vi "AutoRun.vi"() -> ()   [LabVIEW 2013]
uses:
  resultShow.vi
panel:
  in  "布尔":bool
  out "毫秒计时值":u32
  in  "stepMotor/ECU":string
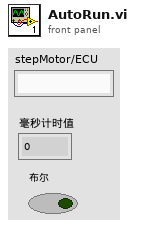
[diagram p1: front panel]
types:
  T1 = cluster{"takesTime":refnum<vi>, "userStatus":refnum<vi>, "userName":refnum<vi>, "connectionMode":refnum<vi>, "productsName":refnum<vi>, "rigStatus":refnum<vi>, "管柱码":refnum<vi>, "上序状态":refnum<vi>}
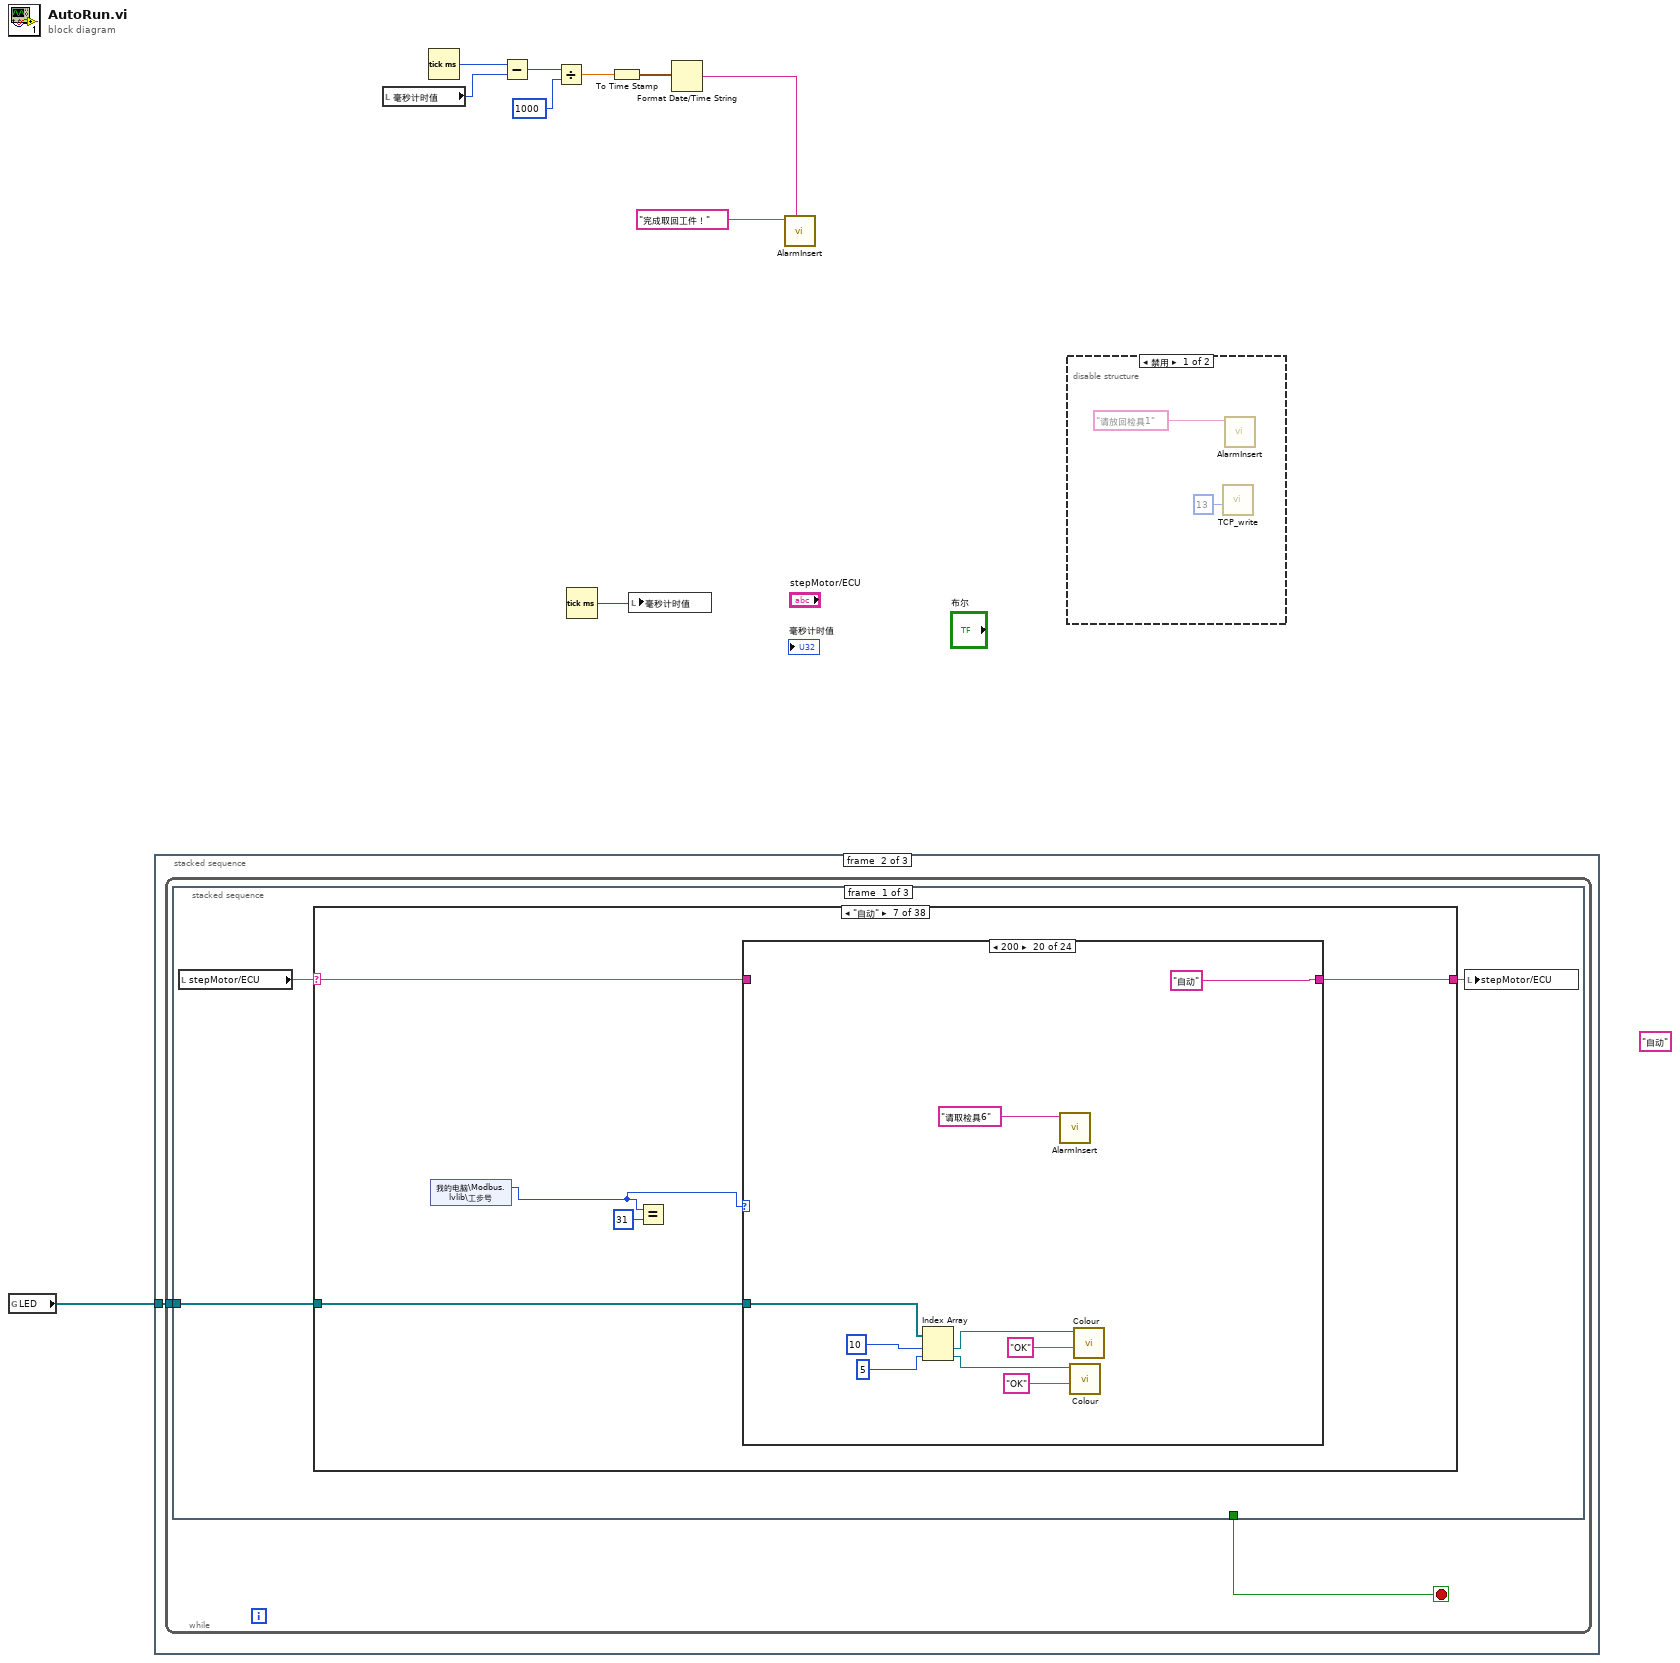
[diagram p0: block diagram]
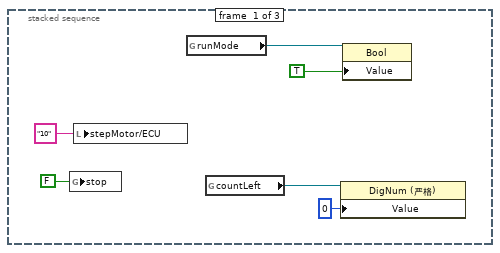
[diagram p3: hidden frame]
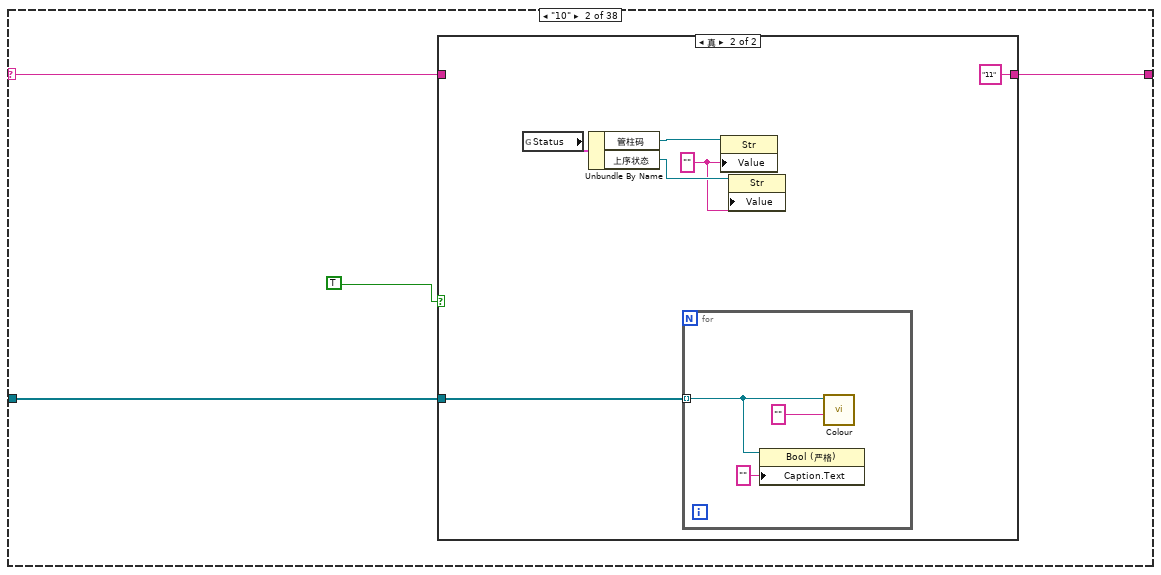
[diagram p5: hidden frame]
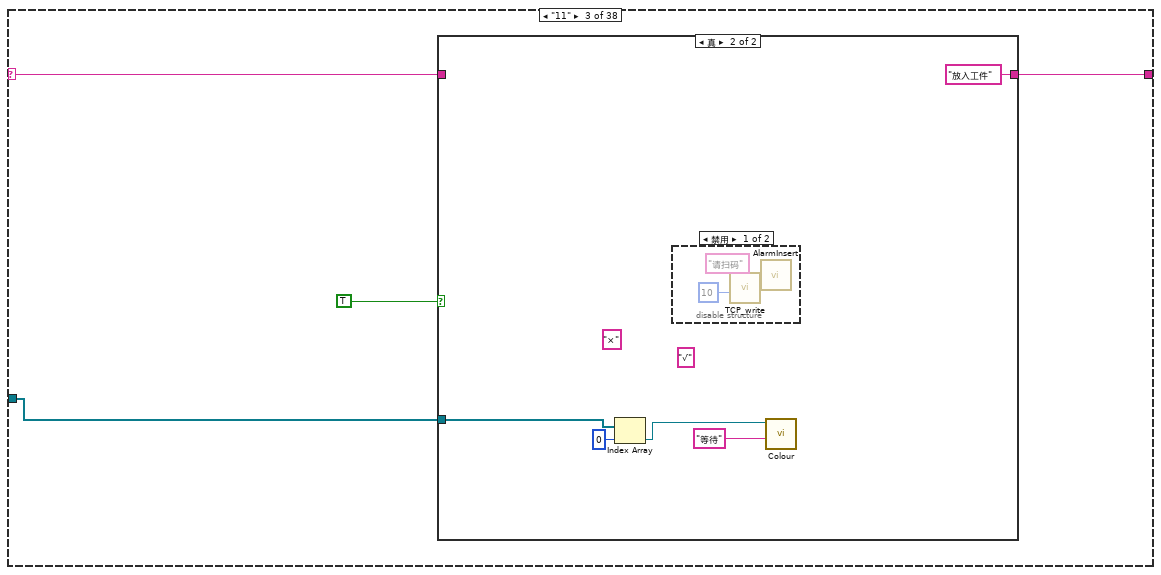
[diagram p7: hidden frame]
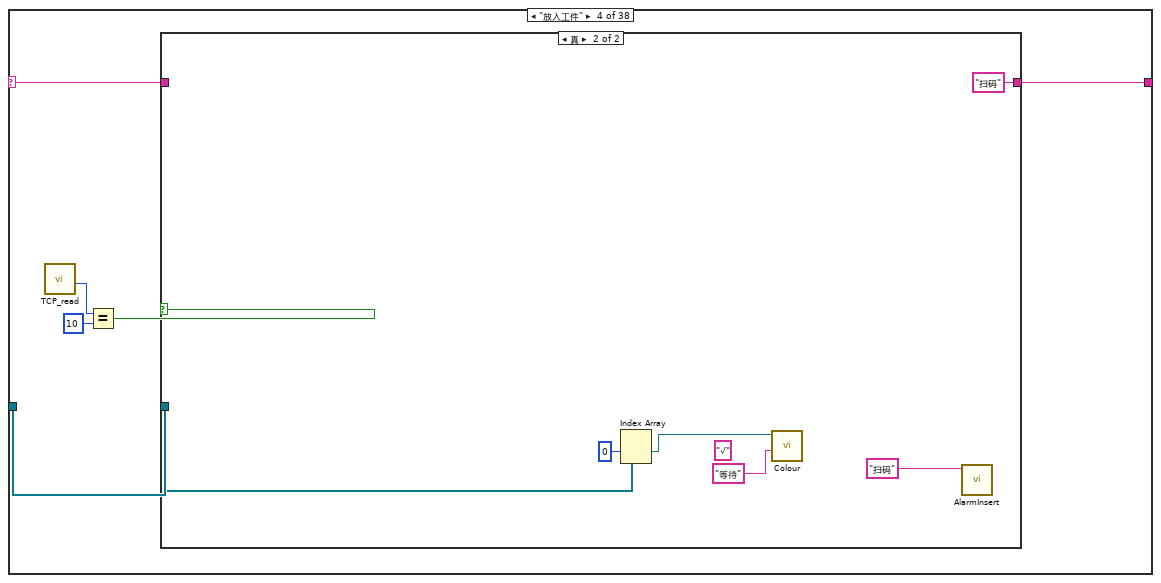
[diagram p10: hidden frame]
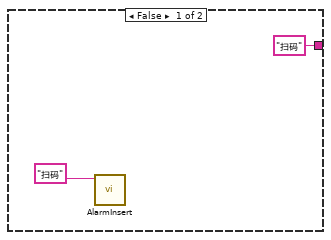
[diagram p11: hidden frame]
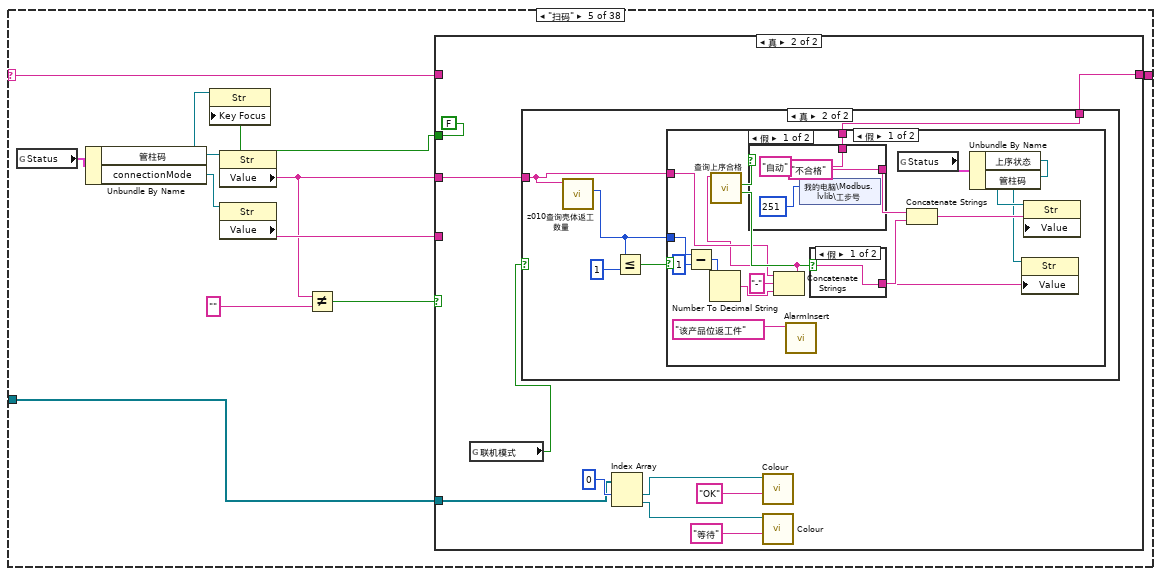
[diagram p12: hidden frame]
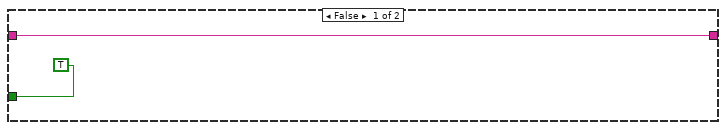
[diagram p13: hidden frame]
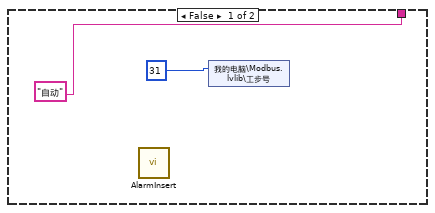
[diagram p14: hidden frame]
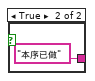
[diagram p15: hidden frame]
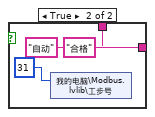
[diagram p16: hidden frame]
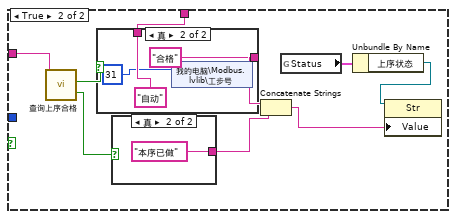
[diagram p17: hidden frame]
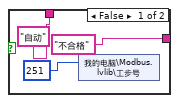
[diagram p19: hidden frame]
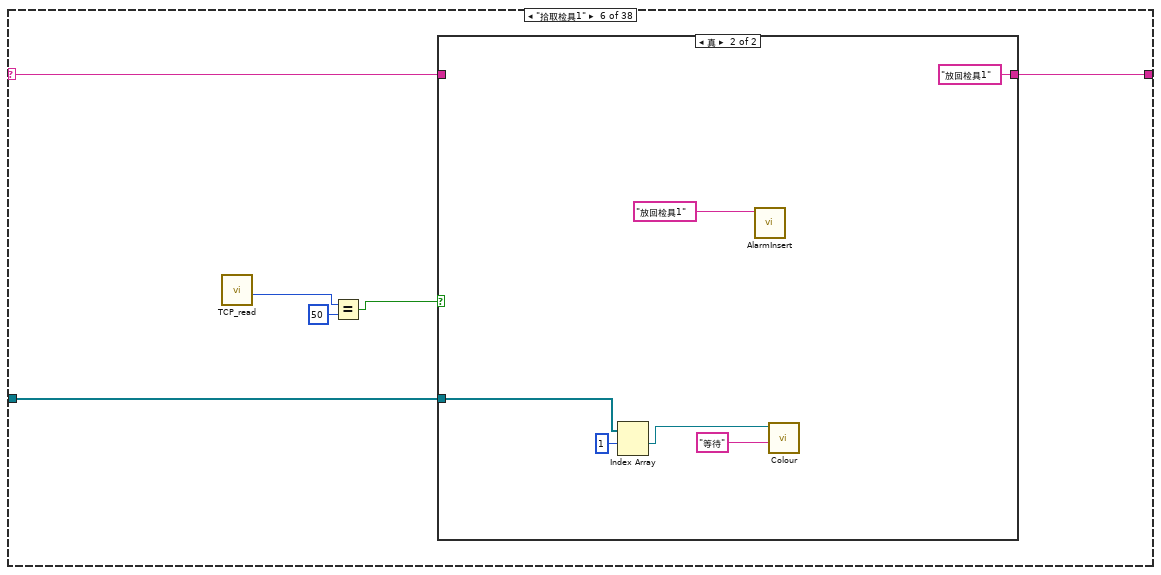
[diagram p20: hidden frame]
diagram:
  (unwired) "自动"
  n1 = global read "resultShow.vi" "LED"() -> (w10:refnum<vi>[])
  n2 = stacked-sequence {
    tunnel: w10 -> [_ w17 _]
    frame #0 {
      n3 = global write "全局 3.vi" "stop"(FALSE ("布尔 2")) -> ()
      n4 = local write "stepMotor/ECU"("10" ("step")) -> ()
      n5 = global read "resultShow.vi" "runMode"() -> (w13:refnum<vi>)
      n6 = global read "resultShow.vi" "countLeft"() -> (w11:refnum<vi>)
      n7 = property class="DigNum (严格)"(reference=w11, "Value"=u32 0 ("值")) -> ()  [unwired: 1 in, 2 out]
      n8 = property class="Bool"(reference=w13, "Value"=TRUE ("m")) -> ()  [unwired: 1 in, 2 out]
    }
    frame #1 {
      n9 = while {
        tunnel: w17 -> [w18]
        stop <- w19 stop-if-true
        n10 = stacked-sequence {
          tunnel: [_ _ w860] -> w19
          tunnel: w18 -> [w21 _ _]
          frame #0 {
            n11 = local read "stepMotor/ECU"() -> (w20:string)
            n12 = case shown="\"自动\"" w20 {
              selector: w20 -> [w23 w26 w40 w51 w72 w137 w149 w331 w347 w363 w381 w397 w413 w429 w445 w461 w477 w493 w509 w525 w541 w557 w573 w589 w605 w621 w637 w653 w669 w685 w701 w717 w733 w749 w765 w781 w795 w823]
              tunnel: [w23 w27 w41 w49 w71 w138 w150 w329 w345 w361 w382 w398 w414 w430 w446 w462 w478 w494 w510 w526 w542 w558 w574 w590 w606 w622 w638 w654 w670 w686 w702 w718 w734 w750 w766 w782 w796 w824] -> w22
              tunnel: w21 -> [_ w25 w39 w50 w73 w133 w147 w330 w346 w362 w377 w393 w409 w425 w441 w457 w473 w489 w505 w521 w537 w553 w569 w585 w601 w617 w633 w649 w665 w681 w697 w713 w729 w745 w761 w777 w794 w819]
              frame "假", Default {
              }
              frame "10" {
                n13 = case shown="真" TRUE {
                  tunnel: [w28 "11"] -> w27
                  tunnel: w26 -> [w28 _]
                  tunnel: w25 -> [_ w33]
                  frame False {
                  }
                  frame True {
                    w29 = ""
                    n14 = global read "resultShow.vi" "Status"() -> (w32:T1)
                    n15 = Unbundle By Name(w32) -> ("管柱码"=w31:refnum<vi>, "上序状态"=w30:refnum<vi>)
                    n16 = for {
                      tunnel: w33 -> [w36] mode=indexing
                      n17 = property class="Bool (严格)"(reference=w36, "Caption.Text"="" ("标题.文本")) -> ()  [unwired: 1 in, 2 out]
                      n18 = call "Colour.vi"("result"="" ("元素"), "colourRef"=w36) -> ()  [unwired: 9 in, 1 out]
                    }
                    n19 = property class="Str"(reference=w31, "Value"=w29) -> ()  [unwired: 1 in, 2 out]
                    n20 = property class="Str"(reference=w30, "Value"=w29) -> ()  [unwired: 1 in, 2 out]
                  }
                }
              }
              frame "11" {
                n21 = case shown="真" TRUE {
                  tunnel: [w42 "放入工件"] -> w41
                  tunnel: w40 -> [w42 _]
                  tunnel: w39 -> [_ w43]
                  frame False {
                  }
                  frame True {
                    (unwired) "×" ("元素")
                    (unwired) "√" ("元素")
                    n22 = Index Array(array=w43, index=0 ("索引")) -> (element=w45:refnum<vi>)
                    n23 = disable-structure shown="禁用" {
                      frame Disabled {
                        (unwired) "请扫码" ("消息名")
                        n24 = call "TCP_write.vi"("写入数据"=i8 10) -> ()  [unwired: 11 in]
                        n25 = call "AlarmInsert.vi"() -> ()  [unwired: 12 in]
                      }
                      frame Enabled {
                      }
                    }
                    n26 = call "Colour.vi"("result"="等待" ("元素"), "colourRef"=w45) -> ()  [unwired: 9 in, 1 out]
                  }
                }
              }
              frame "放入工件" {
                n27 = call "TCP_read.vi"() -> ("元素"=w52:u8)  [unwired: 10 in, 1 out]
                n28 = Equal?(x=w52, y=i8 10) -> (x = y?=w54:bool)
                n29 = case shown="真" w54 {
                  tunnel: ["扫码" "扫码"] -> w49
                  tunnel: w51 -> [_ _]
                  tunnel: w50 -> [_ w59]
                  frame False {
                    n30 = call "AlarmInsert.vi"("消息名"="扫码" ("string_5")) -> ()  [unwired: 11 in]
                  }
                  frame True {
                    (unwired) "√" ("元素")
                    n31 = Index Array(array=w59, index #1=0 ("索引")) -> (element #1=w61:refnum<vi>)  [unwired: 1 in, 1 out]
                    n32 = call "Colour.vi"("result"="等待" ("元素"), "colourRef"=w61) -> ()  [unwired: 9 in, 1 out]
                    n33 = call "AlarmInsert.vi"("消息名"="扫码" ("string_5")) -> ()  [unwired: 11 in]
                  }
                }
              }
              frame "扫码" {
                n34 = global read "resultShow.vi" "Status"() -> (w70:T1)
                n35 = Unbundle By Name(w70) -> ("管柱码"=w68:refnum<vi>, "connectionMode"=w65:refnum<vi>)
                n36 = property class="Str"(reference=w68) -> ("Value"=w63:string)  [unwired: 1 in, 2 out]
                n37 = property class="Str"(reference=w65) -> ("Value"=w64:string)  [unwired: 1 in, 2 out]
                n38 = Not Equal?(x=w63, y="") -> (x != y?=w67:bool)
                n39 = case shown="真" w67 {
                  tunnel: [w75 w76] -> w71
                  tunnel: w72 -> [w75 _]
                  tunnel: w73 -> [_ w82]
                  tunnel: [TRUE FALSE] -> w66
                  tunnel: w64 -> [_ _]
                  tunnel: w63 -> [_ w78]
                  frame False {
                  }
                  frame True {
                    n40 = global read "resultShow.vi" "联机模式"() -> (w77:bool)
                    n41 = case shown="真" w77 {
                      tunnel: w78 -> [_ w90]
                      tunnel: ["自动" ("消息名") w88] -> w76
                      frame False {
                        n42 = call "AlarmInsert.vi"() -> ()  [unwired: 12 in]
                        n43 = shared-variable "我的电脑\\Modbus.lvlib\\工步号"(i8 31 ("写入数据")) -> ()  [unwired: 1 in, 1 out]
                      }
                      frame True {
                        n44 = call "z010查询壳体返工数量.vi"("转向器总成ID"=w90) -> ("Rows Fetched"=w89:i32)  [unwired: 8 in, 2 out]
                        n45 = Less Or Equal?(x=w89, y=1) -> (x <= y?=w91:bool)
                        n46 = case shown="假" w91 {
                          tunnel: w90 -> [w96 w125]
                          tunnel: w89 -> [w101 _]
                          tunnel: [w93 w117] -> w88
                          frame False {
                            n47 = Subtract(x=w101, y=1) -> (x-y=w99:i32)
                            n48 = Number To Decimal String ("数值至十进制数字符串转换")(number=w99) -> (decimal integer string=w98:string)  [unwired: 1 in]
                            n49 = Concatenate Strings(w96, "-" ("字符串"), w98) -> (w94:string)
                            n50 = call "查询上序合格.vi"("产品ID"=w94) -> ("本序已做"=w107:bool, "上序合格"=w108:bool)  [unwired: 8 in, 1 out]
                            n51 = case shown="假" w108 {
                              tunnel: ["不合格" "合格"] -> w104
                              tunnel: ["自动" ("string_5") "自动"] -> w93
                              frame False {
                                n52 = shared-variable "我的电脑\\Modbus.lvlib\\工步号"(251 ("写入数据")) -> ()  [unwired: 1 in, 1 out]
                              }
                              frame True {
                                n53 = shared-variable "我的电脑\\Modbus.lvlib\\工步号"(i8 31 ("写入数据")) -> ()  [unwired: 1 in, 1 out]
                              }
                            }
                            n54 = call "AlarmInsert.vi"("消息名"="该产品位返工件") -> ()  [unwired: 11 in]
                            n55 = case shown="假" w107 {
                              tunnel: [_ "本序已做"] -> w103
                              frame False {
                              }
                              frame True {
                              }
                            }
                            n56 = global read "resultShow.vi" "Status"() -> (w106:T1)
                            n57 = Concatenate Strings(w104, w103) -> (w102:string)
                            n58 = Unbundle By Name(w106) -> ("上序状态"=w105:refnum<vi>, "管柱码"=w95:refnum<vi>)
                            n59 = property class="Str"(reference=w95, "Value"=w94) -> ()  [unwired: 1 in, 2 out]
                            n60 = property class="Str"(reference=w105, "Value"=w102) -> ()  [unwired: 1 in, 2 out]
                          }
                          frame True {
                            n61 = call "查询上序合格.vi"("产品ID"=w125) -> ("本序已做"=w123:bool, "上序合格"=w124:bool)  [unwired: 8 in, 1 out]
                            n62 = case shown="真" w124 {
                              tunnel: ["不合格" "合格"] -> w120
                              tunnel: ["自动" "自动" ("string_5")] -> w117
                              frame False {
                                n63 = shared-variable "我的电脑\\Modbus.lvlib\\工步号"(251 ("索引")) -> ()  [unwired: 1 in, 1 out]
                              }
                              frame True {
                                n64 = shared-variable "我的电脑\\Modbus.lvlib\\工步号"(i8 31 ("写入数据")) -> ()  [unwired: 1 in, 1 out]
                              }
                            }
                            n65 = case shown="真" w123 {
                              tunnel: [_ "本序已做"] -> w119
                              frame False {
                              }
                              frame True {
                              }
                            }
                            n66 = Concatenate Strings(w120, w119) -> (w118:string)
                            n67 = global read "resultShow.vi" "Status"() -> (w122:T1)
                            n68 = Unbundle By Name(w122) -> ("上序状态"=w121:refnum<vi>)
                            n69 = property class="Str"(reference=w121, "Value"=w118) -> ()  [unwired: 1 in, 2 out]
                          }
                        }
                      }
                    }
                    n70 = Index Array(array=w82, index #1=0 ("索引")) -> (element #1=w84:refnum<vi>, element #2=w80:refnum<vi>)  [unwired: 1 in]
                    n71 = call "Colour.vi"("result"="OK" ("元素"), "colourRef"=w84) -> ()  [unwired: 9 in, 1 out]
                    n72 = call "Colour.vi"("result"="等待" ("元素"), "colourRef"=w80) -> ()  [unwired: 9 in, 1 out]
                  }
                }
                n73 = property class="Str"(reference=w68, "Key Focus"=w66) -> ()  [unwired: 1 in, 2 out]
              }
              frame "拾取检具1" {
                n74 = call "TCP_read.vi"() -> ("元素"=w136:u8)  [unwired: 10 in, 1 out]
                n75 = Equal?(x=w136, y=i8 50) -> (x = y?=w134:bool)
                n76 = case shown="真" w134 {
                  tunnel: [w139 "放回检具1"] -> w138
                  tunnel: w137 -> [w139 _]
                  tunnel: w133 -> [_ w141]
                  frame False {
                  }
                  frame True {
                    n77 = Index Array(array=w141, index #1=1 ("索引")) -> (element #1=w143:refnum<vi>)  [unwired: 1 in, 1 out]
                    n78 = call "AlarmInsert.vi"("消息名"="放回检具1" ("string_5")) -> ()  [unwired: 11 in]
                    n79 = call "Colour.vi"("result"="等待" ("元素"), "colourRef"=w143) -> ()  [unwired: 9 in, 1 out]
                  }
                }
              }
              frame "自动" {
                n80 = shared-variable "我的电脑\\Modbus.lvlib\\工步号"() -> (w146:u16)  [unwired: 1 in, 1 out]
                n81 = Equal?(x=w146, y=i8 31) -> ()  [unwired: 1 out]
                n82 = case shown="200" w146 {
                  tunnel: ["自动" "自动" "自动" "自动" "自动" "自动" "自动" "自动" "自动" "自动" "自动" "自动" "自动" "自动" "自动" "自动" "自动" "自动" "自动" "自动" "自动" "10" w313 _] -> w150
                  tunnel: w149 -> [_ _ _ _ _ _ _ _ _ _ _ _ _ _ _ _ _ _ _ _ _ _ _ _]
                  tunnel: w147 -> [_ w154 w163 w172 w186 w189 w203 w211 w220 w226 w235 w240 w248 w254 w263 w272 w281 w287 w296 w305 w311 _ _ w328]
                  frame 0, Default {
                  }
                  frame 31 {
                    n83 = disable-structure shown="禁用" {
                      disable-tunnel: w154 -> [w155 _]
                      frame Disabled {
                        n84 = Index Array(array=w155, index #1=1 ("索引")) -> (element #1=w159:refnum<vi>, element #2=w156:refnum<vi>)  [unwired: 1 in]
                        n85 = call "Colour.vi"("result"="√" ("元素"), "colourRef"=w159) -> ()  [unwired: 9 in, 1 out]
                        n86 = call "Colour.vi"("result"="×" ("元素"), "colourRef"=w156) -> ()  [unwired: 9 in, 1 out]
                      }
                      frame Enabled {
                      }
                    }
                    n87 = call "AlarmInsert.vi"("消息名"="请检查左右拉杆是否在位" ("string_5")) -> ()  [unwired: 11 in]
                  }
                  frame 32 {
                    n88 = disable-structure shown="禁用" {
                      disable-tunnel: w163 -> [w164 _]
                      frame Disabled {
                        n89 = Index Array(array=w164, index #1=1 ("索引")) -> (element #1=w168:refnum<vi>, element #2=w165:refnum<vi>)  [unwired: 1 in]
                        n90 = call "Colour.vi"("result"="√" ("元素"), "colourRef"=w168) -> ()  [unwired: 9 in, 1 out]
                        n91 = call "Colour.vi"("result"="×" ("元素"), "colourRef"=w165) -> ()  [unwired: 9 in, 1 out]
                      }
                      frame Enabled {
                      }
                    }
                    n92 = call "AlarmInsert.vi"("消息名"="请按启动按钮开始" ("string_5")) -> ()  [unwired: 11 in]
                  }
                  frame 33 {
                    n93 = disable-structure shown="禁用" {
                      disable-tunnel: w172 -> [w173 _]
                      frame Disabled {
                        n94 = Index Array(array=w173, index #1=1 ("索引")) -> (element #1=w177:refnum<vi>, element #2=w174:refnum<vi>)  [unwired: 1 in]
                        n95 = call "Colour.vi"("result"="√" ("元素"), "colourRef"=w177) -> ()  [unwired: 9 in, 1 out]
                        n96 = call "Colour.vi"("result"="×" ("元素"), "colourRef"=w174) -> ()  [unwired: 9 in, 1 out]
                      }
                      frame Enabled {
                      }
                    }
                    n97 = call "AlarmInsert.vi"("消息名"="气缸进" ("string_5")) -> ()  [unwired: 11 in]
                  }
                  frame 50 {
                    n98 = Index Array(array=w186, index #1=1 ("索引")) -> (element #1=w183:refnum<vi>, element #2=w180:refnum<vi>)  [unwired: 1 in]
                    n99 = call "AlarmInsert.vi"("消息名"="请取检具1" ("string_5")) -> ()  [unwired: 11 in]
                    n100 = call "Colour.vi"("result"="等待" ("元素"), "colourRef"=w183) -> ()  [unwired: 9 in, 1 out]
                    n101 = call "Colour.vi"("result"="×" ("元素"), "colourRef"=w180) -> ()  [unwired: 9 in, 1 out]
                  }
                  frame 60 {
                    n102 = disable-structure shown="禁用" {
                      disable-tunnel: w189 -> [w195 _]
                      frame Disabled {
                        n103 = Index Array(array=w195, index #1=1 ("索引")) -> (element #1=w193:refnum<vi>, element #2=w190:refnum<vi>)  [unwired: 1 in]
                        n104 = call "Colour.vi"("result"="等待" ("元素"), "colourRef"=w193) -> ()  [unwired: 9 in, 1 out]
                        n105 = call "Colour.vi"("result"="×" ("元素"), "colourRef"=w190) -> ()  [unwired: 9 in, 1 out]
                      }
                      frame Enabled {
                      }
                    }
                    n106 = call "AlarmInsert.vi"("消息名"="请放回检具1" ("string_5")) -> ()  [unwired: 11 in]
                  }
                  frame 70 {
                    n107 = Index Array(array=w203, index #1=1 ("索引")) -> (element #1=w200:refnum<vi>, element #2=w197:refnum<vi>)  [unwired: 1 in]
                    n108 = call "AlarmInsert.vi"("消息名"="请取检具2" ("string_5")) -> ()  [unwired: 11 in]
                    n109 = call "Colour.vi"("result"="OK" ("元素"), "colourRef"=w200) -> ()  [unwired: 9 in, 1 out]
                    n110 = call "Colour.vi"("result"="等待" ("元素"), "colourRef"=w197) -> ()  [unwired: 9 in, 1 out]
                  }
                  frame 80 {
                    n111 = Index Array(array=w211, index #1=1 ("索引")) -> (element #1=w208:refnum<vi>, element #2=w205:refnum<vi>)  [unwired: 1 in]
                    n112 = call "AlarmInsert.vi"("消息名"="请放回检具2" ("string_5")) -> ()  [unwired: 11 in]
                    n113 = call "Colour.vi"("result"="OK" ("元素"), "colourRef"=w208) -> ()  [unwired: 9 in, 1 out]
                    n114 = call "Colour.vi"("result"="等待" ("元素"), "colourRef"=w205) -> ()  [unwired: 9 in, 1 out]
                  }
                  frame 90 {
                    n115 = Index Array(array=w220, index #1=2 ("索引"), index #2=9 ("索引")) -> (element #1=w217:refnum<vi>, element #2=w214:refnum<vi>)
                    n116 = call "AlarmInsert.vi"("消息名"="请取检具9" ("string_5")) -> ()  [unwired: 11 in]
                    n117 = call "Colour.vi"("result"="OK" ("元素"), "colourRef"=w217) -> ()  [unwired: 9 in, 1 out]
                    n118 = call "Colour.vi"("result"="等待" ("元素"), "colourRef"=w214) -> ()  [unwired: 9 in, 1 out]
                  }
                  frame 100 {
                    n119 = Index Array(array=w226, index=9 ("索引")) -> (element=w223:refnum<vi>)
                    n120 = call "AlarmInsert.vi"("消息名"="请放回检具9" ("string_5")) -> ()  [unwired: 11 in]
                    n121 = call "Colour.vi"("result"="等待" ("元素"), "colourRef"=w223) -> ()  [unwired: 9 in, 1 out]
                  }
                  frame 110 {
                    n122 = Index Array(array=w235, index #1=9 ("索引"), index #2=3 ("索引")) -> (element #1=w232:refnum<vi>, element #2=w228:refnum<vi>)
                    n123 = call "AlarmInsert.vi"("消息名"="请取检具3" ("string_5")) -> ()  [unwired: 11 in]
                    n124 = call "Colour.vi"("result"="OK" ("元素"), "colourRef"=w232) -> ()  [unwired: 9 in, 1 out]
                    n125 = call "Colour.vi"("result"="等待" ("元素"), "colourRef"=w228) -> ()  [unwired: 9 in, 1 out]
                  }
                  frame 120 {
                    (unwired) "" ("元素")
                    n126 = Index Array(array=w240, index #1=3 ("索引"), index #2=3 ("索引")) -> ()  [unwired: 2 out]
                    n127 = call "AlarmInsert.vi"("消息名"="请放回检具3" ("string_5")) -> ()  [unwired: 11 in]
                  }
                  frame 130 {
                    n128 = Index Array(array=w248, index #1=3 ("索引")) -> (element #1=w245:refnum<vi>, element #2=w241:refnum<vi>)  [unwired: 1 in]
                    n129 = call "AlarmInsert.vi"("消息名"="请取检具4" ("string_5")) -> ()  [unwired: 11 in]
                    n130 = call "Colour.vi"("result"="OK" ("元素"), "colourRef"=w245) -> ()  [unwired: 9 in, 1 out]
                    n131 = call "Colour.vi"("result"="等待" ("元素"), "colourRef"=w241) -> ()  [unwired: 9 in, 1 out]
                  }
                  frame 140 {
                    n132 = Index Array(array=w254, index #1=4 ("索引")) -> (element #1=w251:refnum<vi>)  [unwired: 1 in, 1 out]
                    n133 = call "AlarmInsert.vi"("消息名"="请放回检具4" ("string_5")) -> ()  [unwired: 11 in]
                    n134 = call "Colour.vi"("result"="等待" ("元素"), "colourRef"=w251) -> ()  [unwired: 9 in, 1 out]
                  }
                  frame 150 {
                    n135 = Index Array(array=w263, index #1=4 ("索引"), index #2=5 ("索引")) -> (element #1=w260:refnum<vi>, element #2=w256:refnum<vi>)
                    n136 = call "AlarmInsert.vi"("消息名"="请取检具5" ("string_5")) -> ()  [unwired: 11 in]
                    n137 = call "Colour.vi"("result"="等待" ("元素"), "colourRef"=w256) -> ()  [unwired: 9 in, 1 out]
                    n138 = call "Colour.vi"("result"="OK" ("元素"), "colourRef"=w260) -> ()  [unwired: 9 in, 1 out]
                  }
                  frame 160 {
                    n139 = Index Array(array=w272, index #1=4 ("索引"), index #2=5 ("索引")) -> (element #1=w269:refnum<vi>, element #2=w265:refnum<vi>)
                    n140 = call "AlarmInsert.vi"("消息名"="请放回检具5" ("string_5")) -> ()  [unwired: 11 in]
                    n141 = call "Colour.vi"("result"="等待" ("元素"), "colourRef"=w265) -> ()  [unwired: 9 in, 1 out]
                    n142 = call "Colour.vi"("result"="OK" ("元素"), "colourRef"=w269) -> ()  [unwired: 9 in, 1 out]
                  }
                  frame 170 {
                    n143 = Index Array(array=w281, index #1=5 ("索引"), index #2=10 ("索引")) -> (element #1=w278:refnum<vi>, element #2=w274:refnum<vi>)
                    n144 = call "AlarmInsert.vi"("消息名"="请取检具10" ("string_5")) -> ()  [unwired: 11 in]
                    n145 = call "Colour.vi"("result"="等待" ("元素"), "colourRef"=w274) -> ()  [unwired: 9 in, 1 out]
                    n146 = call "Colour.vi"("result"="OK" ("元素"), "colourRef"=w278) -> ()  [unwired: 9 in, 1 out]
                  }
                  frame 180 {
                    n147 = Index Array(array=w287, index #1=10 ("索引")) -> (element #1=w284:refnum<vi>)  [unwired: 1 in, 1 out]
                    n148 = call "AlarmInsert.vi"("消息名"="请放回检具10" ("string_5")) -> ()  [unwired: 11 in]
                    n149 = call "Colour.vi"("result"="等待" ("元素"), "colourRef"=w284) -> ()  [unwired: 9 in, 1 out]
                  }
                  frame 190 {
                    n150 = Index Array(array=w296, index #1=10 ("索引"), index #2=5 ("索引")) -> (element #1=w293:refnum<vi>, element #2=w289:refnum<vi>)
                    n151 = call "AlarmInsert.vi"("消息名"="请取检具6" ("string_5")) -> ()  [unwired: 11 in]
                    n152 = call "Colour.vi"("result"="等待" ("元素"), "colourRef"=w289) -> ()  [unwired: 9 in, 1 out]
                    n153 = call "Colour.vi"("result"="OK" ("元素"), "colourRef"=w293) -> ()  [unwired: 9 in, 1 out]
                  }
                  frame 200 {
                    n154 = Index Array(array=w305, index #1=10 ("索引"), index #2=5 ("索引")) -> (element #1=w302:refnum<vi>, element #2=w298:refnum<vi>)
                    n155 = call "AlarmInsert.vi"("消息名"="请取检具6" ("string_5")) -> ()  [unwired: 11 in]
                    n156 = call "Colour.vi"("result"="OK" ("元素"), "colourRef"=w298) -> ()  [unwired: 9 in, 1 out]
                    n157 = call "Colour.vi"("result"="OK" ("元素"), "colourRef"=w302) -> ()  [unwired: 9 in, 1 out]
                  }
                  frame 210 {
                    n158 = Index Array(array=w311, index #1=5 ("索引"), index #2=5 ("索引")) -> (element #1=w309:refnum<vi>)  [unwired: 1 out]
                    n159 = call "Colour.vi"("result"="OK" ("元素"), "colourRef"=w309) -> ()  [unwired: 9 in, 1 out]
                  }
                  frame 251 {
                  }
                  frame 250 {
                    n160 = stacked-sequence {
                      tunnel: [_ "10"] -> w313
                      frame #0 {
                        w320 = "1"
                        n161 = global read "resultShow.vi" "Status"() -> (w319:T1)
                        n162 = Unbundle By Name(w319) -> ("管柱码"=w318:refnum<vi>, "userName"=w316:refnum<vi>)
                        n163 = property class="Str"(reference=w316) -> ("Value"=w315:string)  [unwired: 1 in, 2 out]
                        n164 = property class="Str"(reference=w318) -> ("Value"=w317:string)  [unwired: 1 in, 2 out]
                        n165 = Build Array(w317, w315, w320, w320) -> (w314:string[])
                        n166 = call "数据库更新.vi"("设备号"="14", "数据"=w314) -> ()  [unwired: 13 in, 1 out]
                      }
                      frame #1 {
                        n167 = shared-variable "我的电脑\\Modbus.lvlib\\工步号"(251) -> ()  [unwired: 1 in, 1 out]
                      }
                    }
                  }
                  frame 51 {
                    n168 = Index Array(array=w328, index=1 ("索引")) -> (element=w325:refnum<vi>)
                    n169 = call "AlarmInsert.vi"("消息名"="请取检具1" ("string_5")) -> ()  [unwired: 11 in]
                    n170 = call "Colour.vi"("result"="等待" ("元素"), "colourRef"=w325) -> ()  [unwired: 9 in, 1 out]
                  }
                }
              }
              frame "放回检具1" {
                n171 = call "TCP_read.vi"() -> ("元素"=w334:u8)  [unwired: 10 in, 1 out]
                n172 = Equal?(x=w334, y=i8 60) -> (x = y?=w332:bool)
                n173 = case shown="真" w332 {
                  tunnel: [w335 "拾取检具2"] -> w329
                  tunnel: w331 -> [w335 _]
                  tunnel: w330 -> [_ w337]
                  frame False {
                  }
                  frame True {
                    n174 = Index Array(array=w337, index #1=2 ("索引")) -> (element #1=w341:refnum<vi>, element #2=w338:refnum<vi>)  [unwired: 1 in]
                    n175 = call "TCP_write.vi"("写入数据"=i8 20) -> ()  [unwired: 11 in]
                    n176 = call "AlarmInsert.vi"("消息名"="拾取检具2" ("string_5")) -> ()  [unwired: 11 in]
                    n177 = call "Colour.vi"("result"="OK" ("元素"), "colourRef"=w341) -> ()  [unwired: 9 in, 1 out]
                    n178 = call "Colour.vi"("result"="等待" ("元素"), "colourRef"=w338) -> ()  [unwired: 9 in, 1 out]
                  }
                }
              }
              frame "拾取检具2" {
                n179 = call "TCP_read.vi"() -> ("元素"=w348:u8)  [unwired: 10 in, 1 out]
                n180 = Equal?(x=w348, y=i8 21) -> (x = y?=w350:bool)
                n181 = case shown="真" w350 {
                  tunnel: [w351 "放回检具2"] -> w345
                  tunnel: w347 -> [w351 _]
                  tunnel: w346 -> [_ w353]
                  frame False {
                  }
                  frame True {
                    n182 = Index Array(array=w353, index #1=2 ("索引")) -> (element #1=w357:refnum<vi>, element #2=w354:refnum<vi>)  [unwired: 1 in]
                    n183 = call "TCP_write.vi"("写入数据"=i8 23) -> ()  [unwired: 11 in]
                    n184 = call "AlarmInsert.vi"("消息名"="放回检具2" ("string_5")) -> ()  [unwired: 11 in]
                    n185 = call "Colour.vi"("result"="√" ("元素"), "colourRef"=w357) -> ()  [unwired: 9 in, 1 out]
                    n186 = call "Colour.vi"("result"="×" ("元素"), "colourRef"=w354) -> ()  [unwired: 9 in, 1 out]
                  }
                }
              }
              frame "放回检具2" {
                n187 = call "TCP_read.vi"() -> ("元素"=w364:u8)  [unwired: 10 in, 1 out]
                n188 = Equal?(x=w364, y=i8 25) -> (x = y?=w366:bool)
                n189 = case shown="真" w366 {
                  tunnel: [w367 "拾取检具3"] -> w361
                  tunnel: w363 -> [w367 _]
                  tunnel: w362 -> [_ w369]
                  frame False {
                  }
                  frame True {
                    n190 = Index Array(array=w369, index #1=3 ("索引")) -> (element #1=w373:refnum<vi>, element #2=w370:refnum<vi>)  [unwired: 1 in]
                    n191 = call "TCP_write.vi"("写入数据"=i8 30) -> ()  [unwired: 11 in]
                    n192 = call "AlarmInsert.vi"("消息名"="拾取检具3" ("string_5")) -> ()  [unwired: 11 in]
                    n193 = call "Colour.vi"("result"="√" ("元素"), "colourRef"=w373) -> ()  [unwired: 9 in, 1 out]
                    n194 = call "Colour.vi"("result"="×" ("元素"), "colourRef"=w370) -> ()  [unwired: 9 in, 1 out]
                  }
                }
              }
              frame "拾取检具3" {
                n195 = call "TCP_read.vi"() -> ("元素"=w380:u8)  [unwired: 10 in, 1 out]
                n196 = Equal?(x=w380, y=i8 31) -> (x = y?=w378:bool)
                n197 = case shown="真" w378 {
                  tunnel: [w383 "放回检具3"] -> w382
                  tunnel: w381 -> [w383 _]
                  tunnel: w377 -> [_ w385]
                  frame False {
                  }
                  frame True {
                    n198 = Index Array(array=w385, index #1=3 ("索引")) -> (element #1=w389:refnum<vi>, element #2=w386:refnum<vi>)  [unwired: 1 in]
                    n199 = call "TCP_write.vi"("写入数据"=i8 33) -> ()  [unwired: 11 in]
                    n200 = call "AlarmInsert.vi"("消息名"="放回检具3" ("string_5")) -> ()  [unwired: 11 in]
                    n201 = call "Colour.vi"("result"="√" ("元素"), "colourRef"=w389) -> ()  [unwired: 9 in, 1 out]
                    n202 = call "Colour.vi"("result"="×" ("元素"), "colourRef"=w386) -> ()  [unwired: 9 in, 1 out]
                  }
                }
              }
              frame "放回检具3" {
                n203 = call "TCP_read.vi"() -> ("元素"=w396:u8)  [unwired: 10 in, 1 out]
                n204 = Equal?(x=w396, y=i8 35) -> (x = y?=w394:bool)
                n205 = case shown="真" w394 {
                  tunnel: [w399 "拾取检具4"] -> w398
                  tunnel: w397 -> [w399 _]
                  tunnel: w393 -> [_ w401]
                  frame False {
                  }
                  frame True {
                    n206 = Index Array(array=w401, index #1=4 ("索引")) -> (element #1=w405:refnum<vi>, element #2=w402:refnum<vi>)  [unwired: 1 in]
                    n207 = call "TCP_write.vi"("写入数据"=i8 40) -> ()  [unwired: 11 in]
                    n208 = call "AlarmInsert.vi"("消息名"="拾取检具4" ("string_5")) -> ()  [unwired: 11 in]
                    n209 = call "Colour.vi"("result"="√" ("元素"), "colourRef"=w405) -> ()  [unwired: 9 in, 1 out]
                    n210 = call "Colour.vi"("result"="×" ("元素"), "colourRef"=w402) -> ()  [unwired: 9 in, 1 out]
                  }
                }
              }
              frame "拾取检具4" {
                n211 = call "TCP_read.vi"() -> ("元素"=w412:u8)  [unwired: 10 in, 1 out]
                n212 = Equal?(x=w412, y=i8 41) -> (x = y?=w410:bool)
                n213 = case shown="真" w410 {
                  tunnel: [w415 "放回检具4"] -> w414
                  tunnel: w413 -> [w415 _]
                  tunnel: w409 -> [_ w417]
                  frame False {
                  }
                  frame True {
                    n214 = Index Array(array=w417, index #1=4 ("索引")) -> (element #1=w421:refnum<vi>, element #2=w418:refnum<vi>)  [unwired: 1 in]
                    n215 = call "TCP_write.vi"("写入数据"=i8 43) -> ()  [unwired: 11 in]
                    n216 = call "AlarmInsert.vi"("消息名"="放回检具4" ("string_5")) -> ()  [unwired: 11 in]
                    n217 = call "Colour.vi"("result"="√" ("元素"), "colourRef"=w421) -> ()  [unwired: 9 in, 1 out]
                    n218 = call "Colour.vi"("result"="×" ("元素"), "colourRef"=w418) -> ()  [unwired: 9 in, 1 out]
                  }
                }
              }
              frame "放回检具4" {
                n219 = call "TCP_read.vi"() -> ("元素"=w428:u8)  [unwired: 10 in, 1 out]
                n220 = Equal?(x=w428, y=i8 45) -> (x = y?=w426:bool)
                n221 = case shown="真" w426 {
                  tunnel: [w431 "拾取检具5"] -> w430
                  tunnel: w429 -> [w431 _]
                  tunnel: w425 -> [_ w433]
                  frame False {
                  }
                  frame True {
                    n222 = Index Array(array=w433, index #1=5 ("索引")) -> (element #1=w437:refnum<vi>, element #2=w434:refnum<vi>)  [unwired: 1 in]
                    n223 = call "TCP_write.vi"("写入数据"=i8 50) -> ()  [unwired: 11 in]
                    n224 = call "AlarmInsert.vi"("消息名"="拾取检具5" ("string_5")) -> ()  [unwired: 11 in]
                    n225 = call "Colour.vi"("result"="√" ("元素"), "colourRef"=w437) -> ()  [unwired: 9 in, 1 out]
                    n226 = call "Colour.vi"("result"="×" ("元素"), "colourRef"=w434) -> ()  [unwired: 9 in, 1 out]
                  }
                }
              }
              frame "拾取检具5" {
                n227 = call "TCP_read.vi"() -> ("元素"=w444:u8)  [unwired: 10 in, 1 out]
                n228 = Equal?(x=w444, y=i8 51) -> (x = y?=w442:bool)
                n229 = case shown="真" w442 {
                  tunnel: [w447 "放回检具5"] -> w446
                  tunnel: w445 -> [w447 _]
                  tunnel: w441 -> [_ w449]
                  frame False {
                  }
                  frame True {
                    n230 = Index Array(array=w449, index #1=5 ("索引")) -> (element #1=w453:refnum<vi>, element #2=w450:refnum<vi>)  [unwired: 1 in]
                    n231 = call "TCP_write.vi"("写入数据"=i8 53) -> ()  [unwired: 11 in]
                    n232 = call "AlarmInsert.vi"("消息名"="放回检具5" ("string_5")) -> ()  [unwired: 11 in]
                    n233 = call "Colour.vi"("result"="√" ("元素"), "colourRef"=w453) -> ()  [unwired: 9 in, 1 out]
                    n234 = call "Colour.vi"("result"="×" ("元素"), "colourRef"=w450) -> ()  [unwired: 9 in, 1 out]
                  }
                }
              }
              frame "放回检具5" {
                n235 = call "TCP_read.vi"() -> ("元素"=w460:u8)  [unwired: 10 in, 1 out]
                n236 = Equal?(x=w460, y=i8 55) -> (x = y?=w458:bool)
                n237 = case shown="真" w458 {
                  tunnel: [w463 "拾取检具6"] -> w462
                  tunnel: w461 -> [w463 _]
                  tunnel: w457 -> [_ w465]
                  frame False {
                  }
                  frame True {
                    n238 = Index Array(array=w465, index #1=6 ("索引")) -> (element #1=w469:refnum<vi>, element #2=w466:refnum<vi>)  [unwired: 1 in]
                    n239 = call "TCP_write.vi"("写入数据"=i8 60) -> ()  [unwired: 11 in]
                    n240 = call "AlarmInsert.vi"("消息名"="拾取检具6" ("string_5")) -> ()  [unwired: 11 in]
                    n241 = call "Colour.vi"("result"="√" ("元素"), "colourRef"=w469) -> ()  [unwired: 9 in, 1 out]
                    n242 = call "Colour.vi"("result"="×" ("元素"), "colourRef"=w466) -> ()  [unwired: 9 in, 1 out]
                  }
                }
              }
              frame "拾取检具6" {
                n243 = call "TCP_read.vi"() -> ("元素"=w476:u8)  [unwired: 10 in, 1 out]
                n244 = Equal?(x=w476, y=i8 61) -> (x = y?=w474:bool)
                n245 = case shown="真" w474 {
                  tunnel: [w479 "放回检具6"] -> w478
                  tunnel: w477 -> [w479 _]
                  tunnel: w473 -> [_ w481]
                  frame False {
                  }
                  frame True {
                    n246 = Index Array(array=w481, index #1=6 ("索引")) -> (element #1=w485:refnum<vi>, element #2=w482:refnum<vi>)  [unwired: 1 in]
                    n247 = call "TCP_write.vi"("写入数据"=i8 63) -> ()  [unwired: 11 in]
                    n248 = call "AlarmInsert.vi"("消息名"="放回检具6" ("string_5")) -> ()  [unwired: 11 in]
                    n249 = call "Colour.vi"("result"="√" ("元素"), "colourRef"=w485) -> ()  [unwired: 9 in, 1 out]
                    n250 = call "Colour.vi"("result"="×" ("元素"), "colourRef"=w482) -> ()  [unwired: 9 in, 1 out]
                  }
                }
              }
              frame "放回检具6" {
                n251 = call "TCP_read.vi"() -> ("元素"=w492:u8)  [unwired: 10 in, 1 out]
                n252 = Equal?(x=w492, y=i8 65) -> (x = y?=w490:bool)
                n253 = case shown="真" w490 {
                  tunnel: [w495 "拾取检具7"] -> w494
                  tunnel: w493 -> [w495 _]
                  tunnel: w489 -> [_ w497]
                  frame False {
                  }
                  frame True {
                    n254 = Index Array(array=w497, index #1=7 ("索引")) -> (element #1=w501:refnum<vi>, element #2=w498:refnum<vi>)  [unwired: 1 in]
                    n255 = call "TCP_write.vi"("写入数据"=i8 70) -> ()  [unwired: 11 in]
                    n256 = call "AlarmInsert.vi"("消息名"="拾取检具7" ("string_5")) -> ()  [unwired: 11 in]
                    n257 = call "Colour.vi"("result"="√" ("元素"), "colourRef"=w501) -> ()  [unwired: 9 in, 1 out]
                    n258 = call "Colour.vi"("result"="×" ("元素"), "colourRef"=w498) -> ()  [unwired: 9 in, 1 out]
                  }
                }
              }
              frame "拾取检具7" {
                n259 = call "TCP_read.vi"() -> ("元素"=w508:u8)  [unwired: 10 in, 1 out]
                n260 = Equal?(x=w508, y=i8 71) -> (x = y?=w506:bool)
                n261 = case shown="真" w506 {
                  tunnel: [w511 "放回检具7"] -> w510
                  tunnel: w509 -> [w511 _]
                  tunnel: w505 -> [_ w513]
                  frame False {
                  }
                  frame True {
                    n262 = Index Array(array=w513, index #1=7 ("索引")) -> (element #1=w517:refnum<vi>, element #2=w514:refnum<vi>)  [unwired: 1 in]
                    n263 = call "TCP_write.vi"("写入数据"=i8 73) -> ()  [unwired: 11 in]
                    n264 = call "AlarmInsert.vi"("消息名"="放回检具7" ("string_5")) -> ()  [unwired: 11 in]
                    n265 = call "Colour.vi"("result"="√" ("元素"), "colourRef"=w517) -> ()  [unwired: 9 in, 1 out]
                    n266 = call "Colour.vi"("result"="×" ("元素"), "colourRef"=w514) -> ()  [unwired: 9 in, 1 out]
                  }
                }
              }
              frame "放回检具7" {
                n267 = call "TCP_read.vi"() -> ("元素"=w524:u8)  [unwired: 10 in, 1 out]
                n268 = Equal?(x=w524, y=i8 75) -> (x = y?=w522:bool)
                n269 = case shown="真" w522 {
                  tunnel: [w527 "拾取检具8"] -> w526
                  tunnel: w525 -> [w527 _]
                  tunnel: w521 -> [_ w529]
                  frame False {
                  }
                  frame True {
                    n270 = Index Array(array=w529, index #1=8 ("索引")) -> (element #1=w533:refnum<vi>, element #2=w530:refnum<vi>)  [unwired: 1 in]
                    n271 = call "TCP_write.vi"("写入数据"=i8 80) -> ()  [unwired: 11 in]
                    n272 = call "AlarmInsert.vi"("消息名"="拾取检具8" ("string_5")) -> ()  [unwired: 11 in]
                    n273 = call "Colour.vi"("result"="√" ("元素"), "colourRef"=w533) -> ()  [unwired: 9 in, 1 out]
                    n274 = call "Colour.vi"("result"="×" ("元素"), "colourRef"=w530) -> ()  [unwired: 9 in, 1 out]
                  }
                }
              }
              frame "拾取检具8" {
                n275 = call "TCP_read.vi"() -> ("元素"=w540:u8)  [unwired: 10 in, 1 out]
                n276 = Equal?(x=w540, y=i8 81) -> (x = y?=w538:bool)
                n277 = case shown="真" w538 {
                  tunnel: [w543 "放回检具8"] -> w542
                  tunnel: w541 -> [w543 _]
                  tunnel: w537 -> [_ w545]
                  frame False {
                  }
                  frame True {
                    n278 = Index Array(array=w545, index #1=8 ("索引")) -> (element #1=w549:refnum<vi>, element #2=w546:refnum<vi>)  [unwired: 1 in]
                    n279 = call "TCP_write.vi"("写入数据"=i8 83) -> ()  [unwired: 11 in]
                    n280 = call "AlarmInsert.vi"("消息名"="放回检具8" ("string_5")) -> ()  [unwired: 11 in]
                    n281 = call "Colour.vi"("result"="√" ("元素"), "colourRef"=w549) -> ()  [unwired: 9 in, 1 out]
                    n282 = call "Colour.vi"("result"="×" ("元素"), "colourRef"=w546) -> ()  [unwired: 9 in, 1 out]
                  }
                }
              }
              frame "放回检具8" {
                n283 = call "TCP_read.vi"() -> ("元素"=w556:u8)  [unwired: 10 in, 1 out]
                n284 = Equal?(x=w556, y=i8 85) -> (x = y?=w554:bool)
                n285 = case shown="真" w554 {
                  tunnel: [w559 "拾取检具9"] -> w558
                  tunnel: w557 -> [w559 _]
                  tunnel: w553 -> [_ w561]
                  frame False {
                  }
                  frame True {
                    n286 = Index Array(array=w561, index #1=9 ("索引")) -> (element #1=w565:refnum<vi>, element #2=w562:refnum<vi>)  [unwired: 1 in]
                    n287 = call "TCP_write.vi"("写入数据"=i8 86) -> ()  [unwired: 11 in]
                    n288 = call "AlarmInsert.vi"("消息名"="拾取检具9" ("string_5")) -> ()  [unwired: 11 in]
                    n289 = call "Colour.vi"("result"="√" ("元素"), "colourRef"=w565) -> ()  [unwired: 9 in, 1 out]
                    n290 = call "Colour.vi"("result"="×" ("元素"), "colourRef"=w562) -> ()  [unwired: 9 in, 1 out]
                  }
                }
              }
              frame "拾取检具9" {
                n291 = call "TCP_read.vi"() -> ("元素"=w572:u8)  [unwired: 10 in, 1 out]
                n292 = Equal?(x=w572, y=i8 87) -> (x = y?=w570:bool)
                n293 = case shown="真" w570 {
                  tunnel: [w575 "放回检具9"] -> w574
                  tunnel: w573 -> [w575 _]
                  tunnel: w569 -> [_ w577]
                  frame False {
                  }
                  frame True {
                    n294 = Index Array(array=w577, index #1=9 ("索引")) -> (element #1=w581:refnum<vi>, element #2=w578:refnum<vi>)  [unwired: 1 in]
                    n295 = call "TCP_write.vi"("写入数据"=i8 88) -> ()  [unwired: 11 in]
                    n296 = call "AlarmInsert.vi"("消息名"="放回检具9" ("string_5")) -> ()  [unwired: 11 in]
                    n297 = call "Colour.vi"("result"="√" ("元素"), "colourRef"=w581) -> ()  [unwired: 9 in, 1 out]
                    n298 = call "Colour.vi"("result"="×" ("元素"), "colourRef"=w578) -> ()  [unwired: 9 in, 1 out]
                  }
                }
              }
              frame "放回检具9" {
                n299 = call "TCP_read.vi"() -> ("元素"=w588:u8)  [unwired: 10 in, 1 out]
                n300 = Equal?(x=w588, y=i8 89) -> (x = y?=w586:bool)
                n301 = case shown="真" w586 {
                  tunnel: [w591 "拾取检具10"] -> w590
                  tunnel: w589 -> [w591 _]
                  tunnel: w585 -> [_ w593]
                  frame False {
                  }
                  frame True {
                    n302 = Index Array(array=w593, index #1=10 ("索引")) -> (element #1=w597:refnum<vi>, element #2=w594:refnum<vi>)  [unwired: 1 in]
                    n303 = call "TCP_write.vi"("写入数据"=i8 90) -> ()  [unwired: 11 in]
                    n304 = call "AlarmInsert.vi"("消息名"="拾取检具10" ("string_5")) -> ()  [unwired: 11 in]
                    n305 = call "Colour.vi"("result"="√" ("元素"), "colourRef"=w597) -> ()  [unwired: 9 in, 1 out]
                    n306 = call "Colour.vi"("result"="×" ("元素"), "colourRef"=w594) -> ()  [unwired: 9 in, 1 out]
                  }
                }
              }
              frame "拾取检具10" {
                n307 = call "TCP_read.vi"() -> ("元素"=w604:u8)  [unwired: 10 in, 1 out]
                n308 = Equal?(x=w604, y=i8 91) -> (x = y?=w602:bool)
                n309 = case shown="真" w602 {
                  tunnel: [w607 "放回检具10"] -> w606
                  tunnel: w605 -> [w607 _]
                  tunnel: w601 -> [_ w609]
                  frame False {
                  }
                  frame True {
                    n310 = Index Array(array=w609, index #1=10 ("索引")) -> (element #1=w613:refnum<vi>, element #2=w610:refnum<vi>)  [unwired: 1 in]
                    n311 = call "TCP_write.vi"("写入数据"=i8 92) -> ()  [unwired: 11 in]
                    n312 = call "AlarmInsert.vi"("消息名"="放回检具10" ("string_5")) -> ()  [unwired: 11 in]
                    n313 = call "Colour.vi"("result"="√" ("元素"), "colourRef"=w613) -> ()  [unwired: 9 in, 1 out]
                    n314 = call "Colour.vi"("result"="×" ("元素"), "colourRef"=w610) -> ()  [unwired: 9 in, 1 out]
                  }
                }
              }
              frame "放回检具10" {
                n315 = call "TCP_read.vi"() -> ("元素"=w620:u8)  [unwired: 10 in, 1 out]
                n316 = Equal?(x=w620, y=i8 93) -> (x = y?=w618:bool)
                n317 = case shown="真" w618 {
                  tunnel: [w623 "拾取检具11"] -> w622
                  tunnel: w621 -> [w623 _]
                  tunnel: w617 -> [_ w625]
                  frame False {
                  }
                  frame True {
                    n318 = Index Array(array=w625, index #1=11 ("索引")) -> (element #1=w629:refnum<vi>, element #2=w626:refnum<vi>)  [unwired: 1 in]
                    n319 = call "TCP_write.vi"("写入数据"=i8 94) -> ()  [unwired: 11 in]
                    n320 = call "AlarmInsert.vi"("消息名"="拾取检具11" ("string_5")) -> ()  [unwired: 11 in]
                    n321 = call "Colour.vi"("result"="√" ("元素"), "colourRef"=w629) -> ()  [unwired: 9 in, 1 out]
                    n322 = call "Colour.vi"("result"="×" ("元素"), "colourRef"=w626) -> ()  [unwired: 9 in, 1 out]
                  }
                }
              }
              frame "拾取检具11" {
                n323 = call "TCP_read.vi"() -> ("元素"=w636:u8)  [unwired: 10 in, 1 out]
                n324 = Equal?(x=w636, y=i8 95) -> (x = y?=w634:bool)
                n325 = case shown="真" w634 {
                  tunnel: [w639 "放回检具11"] -> w638
                  tunnel: w637 -> [w639 _]
                  tunnel: w633 -> [_ w641]
                  frame False {
                  }
                  frame True {
                    n326 = Index Array(array=w641, index #1=11 ("索引")) -> (element #1=w645:refnum<vi>, element #2=w642:refnum<vi>)  [unwired: 1 in]
                    n327 = call "TCP_write.vi"("写入数据"=i8 96) -> ()  [unwired: 11 in]
                    n328 = call "AlarmInsert.vi"("消息名"="放回检具11" ("string_5")) -> ()  [unwired: 11 in]
                    n329 = call "Colour.vi"("result"="√" ("元素"), "colourRef"=w645) -> ()  [unwired: 9 in, 1 out]
                    n330 = call "Colour.vi"("result"="×" ("元素"), "colourRef"=w642) -> ()  [unwired: 9 in, 1 out]
                  }
                }
              }
              frame "放回检具11" {
                n331 = call "TCP_read.vi"() -> ("元素"=w652:u8)  [unwired: 10 in, 1 out]
                n332 = Equal?(x=w652, y=i8 97) -> (x = y?=w650:bool)
                n333 = case shown="真" w650 {
                  tunnel: [w655 "拾取检具12"] -> w654
                  tunnel: w653 -> [w655 _]
                  tunnel: w649 -> [_ w657]
                  frame False {
                  }
                  frame True {
                    n334 = Index Array(array=w657, index #1=12 ("索引")) -> (element #1=w661:refnum<vi>, element #2=w658:refnum<vi>)  [unwired: 1 in]
                    n335 = call "TCP_write.vi"("写入数据"=i8 98) -> ()  [unwired: 11 in]
                    n336 = call "AlarmInsert.vi"("消息名"="拾取检具12" ("string_5")) -> ()  [unwired: 11 in]
                    n337 = call "Colour.vi"("result"="√" ("元素"), "colourRef"=w661) -> ()  [unwired: 9 in, 1 out]
                    n338 = call "Colour.vi"("result"="×" ("元素"), "colourRef"=w658) -> ()  [unwired: 9 in, 1 out]
                  }
                }
              }
              frame "拾取检具12" {
                n339 = call "TCP_read.vi"() -> ("元素"=w668:u8)  [unwired: 10 in, 1 out]
                n340 = Equal?(x=w668, y=i8 99) -> (x = y?=w666:bool)
                n341 = case shown="真" w666 {
                  tunnel: [w671 "放回检具12"] -> w670
                  tunnel: w669 -> [w671 _]
                  tunnel: w665 -> [_ w673]
                  frame False {
                  }
                  frame True {
                    n342 = Index Array(array=w673, index #1=12 ("索引")) -> (element #1=w677:refnum<vi>, element #2=w674:refnum<vi>)  [unwired: 1 in]
                    n343 = call "TCP_write.vi"("写入数据"=i8 100) -> ()  [unwired: 11 in]
                    n344 = call "AlarmInsert.vi"("消息名"="放回检具12" ("string_5")) -> ()  [unwired: 11 in]
                    n345 = call "Colour.vi"("result"="√" ("元素"), "colourRef"=w677) -> ()  [unwired: 9 in, 1 out]
                    n346 = call "Colour.vi"("result"="×" ("元素"), "colourRef"=w674) -> ()  [unwired: 9 in, 1 out]
                  }
                }
              }
              frame "放回检具12" {
                n347 = call "TCP_read.vi"() -> ("元素"=w684:u8)  [unwired: 10 in, 1 out]
                n348 = Equal?(x=w684, y=i8 101) -> (x = y?=w682:bool)
                n349 = case shown="真" w682 {
                  tunnel: [w687 "拾取检具13"] -> w686
                  tunnel: w685 -> [w687 _]
                  tunnel: w681 -> [_ w689]
                  frame False {
                  }
                  frame True {
                    n350 = Index Array(array=w689, index #1=13 ("索引")) -> (element #1=w693:refnum<vi>, element #2=w690:refnum<vi>)  [unwired: 1 in]
                    n351 = call "TCP_write.vi"("写入数据"=i8 102) -> ()  [unwired: 11 in]
                    n352 = call "AlarmInsert.vi"("消息名"="拾取检具13" ("string_5")) -> ()  [unwired: 11 in]
                    n353 = call "Colour.vi"("result"="√" ("元素"), "colourRef"=w693) -> ()  [unwired: 9 in, 1 out]
                    n354 = call "Colour.vi"("result"="×" ("元素"), "colourRef"=w690) -> ()  [unwired: 9 in, 1 out]
                  }
                }
              }
              frame "拾取检具13" {
                n355 = call "TCP_read.vi"() -> ("元素"=w700:u8)  [unwired: 10 in, 1 out]
                n356 = Equal?(x=w700, y=i8 103) -> (x = y?=w698:bool)
                n357 = case shown="真" w698 {
                  tunnel: [w703 "放回检具13"] -> w702
                  tunnel: w701 -> [w703 _]
                  tunnel: w697 -> [_ w705]
                  frame False {
                  }
                  frame True {
                    n358 = Index Array(array=w705, index #1=13 ("索引")) -> (element #1=w709:refnum<vi>, element #2=w706:refnum<vi>)  [unwired: 1 in]
                    n359 = call "TCP_write.vi"("写入数据"=i8 104) -> ()  [unwired: 11 in]
                    n360 = call "AlarmInsert.vi"("消息名"="放回检具13" ("string_5")) -> ()  [unwired: 11 in]
                    n361 = call "Colour.vi"("result"="√" ("元素"), "colourRef"=w709) -> ()  [unwired: 9 in, 1 out]
                    n362 = call "Colour.vi"("result"="×" ("元素"), "colourRef"=w706) -> ()  [unwired: 9 in, 1 out]
                  }
                }
              }
              frame "放回检具13" {
                n363 = call "TCP_read.vi"() -> ("元素"=w716:u8)  [unwired: 10 in, 1 out]
                n364 = Equal?(x=w716, y=i8 105) -> (x = y?=w714:bool)
                n365 = case shown="真" w714 {
                  tunnel: [w719 "拾取检具14"] -> w718
                  tunnel: w717 -> [w719 _]
                  tunnel: w713 -> [_ w721]
                  frame False {
                  }
                  frame True {
                    n366 = Index Array(array=w721, index #1=14 ("索引")) -> (element #1=w725:refnum<vi>, element #2=w722:refnum<vi>)  [unwired: 1 in]
                    n367 = call "TCP_write.vi"("写入数据"=i8 106) -> ()  [unwired: 11 in]
                    n368 = call "AlarmInsert.vi"("消息名"="拾取检具14" ("string_5")) -> ()  [unwired: 11 in]
                    n369 = call "Colour.vi"("result"="√" ("元素"), "colourRef"=w725) -> ()  [unwired: 9 in, 1 out]
                    n370 = call "Colour.vi"("result"="×" ("元素"), "colourRef"=w722) -> ()  [unwired: 9 in, 1 out]
                  }
                }
              }
              frame "拾取检具14" {
                n371 = call "TCP_read.vi"() -> ("元素"=w732:u8)  [unwired: 10 in, 1 out]
                n372 = Equal?(x=w732, y=i8 107) -> (x = y?=w730:bool)
                n373 = case shown="真" w730 {
                  tunnel: [w735 "放回检具14"] -> w734
                  tunnel: w733 -> [w735 _]
                  tunnel: w729 -> [_ w737]
                  frame False {
                  }
                  frame True {
                    n374 = Index Array(array=w737, index #1=14 ("索引")) -> (element #1=w741:refnum<vi>, element #2=w738:refnum<vi>)  [unwired: 1 in]
                    n375 = call "TCP_write.vi"("写入数据"=i8 108) -> ()  [unwired: 11 in]
                    n376 = call "AlarmInsert.vi"("消息名"="放回检具14" ("string_5")) -> ()  [unwired: 11 in]
                    n377 = call "Colour.vi"("result"="√" ("元素"), "colourRef"=w741) -> ()  [unwired: 9 in, 1 out]
                    n378 = call "Colour.vi"("result"="×" ("元素"), "colourRef"=w738) -> ()  [unwired: 9 in, 1 out]
                  }
                }
              }
              frame "放回检具14" {
                n379 = call "TCP_read.vi"() -> ("元素"=w748:u8)  [unwired: 10 in, 1 out]
                n380 = Equal?(x=w748, y=i8 109) -> (x = y?=w746:bool)
                n381 = case shown="真" w746 {
                  tunnel: [w751 "拾取检具15"] -> w750
                  tunnel: w749 -> [w751 _]
                  tunnel: w745 -> [_ w753]
                  frame False {
                  }
                  frame True {
                    n382 = Index Array(array=w753, index #1=15 ("索引")) -> (element #1=w757:refnum<vi>, element #2=w754:refnum<vi>)  [unwired: 1 in]
                    n383 = call "TCP_write.vi"("写入数据"=i8 110) -> ()  [unwired: 11 in]
                    n384 = call "AlarmInsert.vi"("消息名"="拾取检具15" ("string_5")) -> ()  [unwired: 11 in]
                    n385 = call "Colour.vi"("result"="√" ("元素"), "colourRef"=w757) -> ()  [unwired: 9 in, 1 out]
                    n386 = call "Colour.vi"("result"="×" ("元素"), "colourRef"=w754) -> ()  [unwired: 9 in, 1 out]
                  }
                }
              }
              frame "拾取检具15" {
                n387 = call "TCP_read.vi"() -> ("元素"=w764:u8)  [unwired: 10 in, 1 out]
                n388 = Equal?(x=w764, y=i8 111) -> (x = y?=w762:bool)
                n389 = case shown="真" w762 {
                  tunnel: [w767 "放回检具15"] -> w766
                  tunnel: w765 -> [w767 _]
                  tunnel: w761 -> [_ w769]
                  frame False {
                  }
                  frame True {
                    n390 = Index Array(array=w769, index #1=15 ("索引")) -> (element #1=w773:refnum<vi>, element #2=w770:refnum<vi>)  [unwired: 1 in]
                    n391 = call "TCP_write.vi"("写入数据"=i8 112) -> ()  [unwired: 11 in]
                    n392 = call "AlarmInsert.vi"("消息名"="放回检具15" ("string_5")) -> ()  [unwired: 11 in]
                    n393 = call "Colour.vi"("result"="√" ("元素"), "colourRef"=w773) -> ()  [unwired: 9 in, 1 out]
                    n394 = call "Colour.vi"("result"="×" ("元素"), "colourRef"=w770) -> ()  [unwired: 9 in, 1 out]
                  }
                }
              }
              frame "放回检具15" {
                n395 = call "TCP_read.vi"() -> ("元素"=w780:u8)  [unwired: 10 in, 1 out]
                n396 = Equal?(x=w780, y=i8 113) -> (x = y?=w778:bool)
                n397 = case shown="真" w778 {
                  tunnel: [w783 "判断是否合格"] -> w782
                  tunnel: w781 -> [w783 _]
                  tunnel: w777 -> [_ w785]
                  frame False {
                  }
                  frame True {
                    n398 = Index Array(array=w785, index #1=16 ("索引")) -> (element #1=w789:refnum<vi>, element #2=w786:refnum<vi>)  [unwired: 1 in]
                    n399 = call "TCP_write.vi"("写入数据"=i8 114) -> ()  [unwired: 11 in]
                    n400 = call "AlarmInsert.vi"("消息名"="判断是否合格" ("string_5")) -> ()  [unwired: 11 in]
                    n401 = call "Colour.vi"("result"="√" ("元素"), "colourRef"=w789) -> ()  [unwired: 9 in, 1 out]
                    n402 = call "Colour.vi"("result"="×" ("元素"), "colourRef"=w786) -> ()  [unwired: 9 in, 1 out]
                  }
                }
              }
              frame "判断是否合格" {
                n403 = call "TCP_read.vi"() -> ("元素"=w793:u8)  [unwired: 10 in, 1 out]
                n404 = case shown="115" w793 {
                  tunnel: [w797 w800 w810 "91"] -> w796
                  tunnel: w795 -> [w797 w800 w810 _]
                  tunnel: w794 -> [_ w802 w811 _]
                  frame Default {
                  }
                  frame 115 {
                    n405 = Index Array(array=w802, index #1=17 ("索引")) -> (element #1=w806:refnum<vi>, element #2=w803:refnum<vi>)  [unwired: 1 in]
                    n406 = global write "全局 3.vi" "总合格状态"("×" ("元素")) -> ()
                    n407 = global write "全局 3.vi" "合格判断"("×" ("元素")) -> ()
                    n408 = call "AlarmInsert.vi"("消息名"="不合格 取出工件" ("string_5")) -> ()  [unwired: 11 in]
                    n409 = call "Colour.vi"("result"="×" ("元素"), "colourRef"=w806) -> ()  [unwired: 9 in, 1 out]
                    n410 = call "Colour.vi"("result"="×" ("元素"), "colourRef"=w803) -> ()  [unwired: 9 in, 1 out]
                  }
                  frame 116 {
                    n411 = Index Array(array=w811, index #1=17 ("索引")) -> (element #1=w813:refnum<vi>, element #2=w816:refnum<vi>)  [unwired: 1 in]
                    n412 = global write "全局 3.vi" "总合格状态"("" ("元素")) -> ()
                    n413 = global write "全局 3.vi" "合格判断"("√" ("元素")) -> ()
                    n414 = call "AlarmInsert.vi"("消息名"="合格 取出工件" ("string_5")) -> ()  [unwired: 11 in]
                    n415 = call "Colour.vi"("result"="√" ("元素"), "colourRef"=w813) -> ()  [unwired: 9 in, 1 out]
                    n416 = call "Colour.vi"("result"="×" ("元素"), "colourRef"=w816) -> ()  [unwired: 9 in, 1 out]
                  }
                  frame 120 {
                  }
                }
              }
              frame "91" {
                n417 = call "TCP_read.vi"() -> ("元素"=w822:u8)  [unwired: 10 in, 1 out]
                n418 = Equal?(x=w822, y=i8 120) -> (x = y?=w820:bool)
                n419 = case shown="真" w820 {
                  tunnel: [w825 "10"] -> w824
                  tunnel: w823 -> [w825 _]
                  tunnel: w819 -> [_ w837]
                  frame False {
                  }
                  frame True {
                    n420 = global read "resultShow.vi" "Status"() -> (w829:T1)
                    n421 = global read "resultShow.vi" "countLeft"() -> (w832:refnum<vi>)
                    n422 = Unbundle By Name(w829) -> ("connectionMode"=w830:refnum<vi>)
                    n423 = Index Array(array=w837, index=18 ("索引")) -> (element=w839:refnum<vi>)
                    n424 = property class="DigNum (严格)"(reference=w832) -> (reference out=w836:refnum<vi>, "Value"=w835:u32)  [unwired: 1 in, 1 out]
                    n425 = property class="Str"(reference=w830) -> ("Value"=w828:string)  [unwired: 1 in, 2 out]
                    n426 = call "Colour.vi"("result"="√" ("元素"), "colourRef"=w839) -> ()  [unwired: 9 in, 1 out]
                    n427 = call "AlarmInsert.vi"("消息名"="完成" ("string_5")) -> ()  [unwired: 11 in]
                    n428 = Increment(x=w835) -> (x+1=w834:u32)
                    n429 = Equal?(x=w828, y="联网") -> (x = y?=w826:bool)
                    n430 = call "TCP_write.vi"("写入数据"=i8 0) -> ()  [unwired: 11 in]
                    n431 = case shown="真" w826 {
                      frame False {
                      }
                      frame True {
                        n432 = call "updateiqual.vi"() -> ()  [unwired: 11 in]
                      }
                    }
                    n433 = property class="DigNum (严格)"(reference=w836, "Value"=w834) -> ()  [unwired: 1 in, 2 out]
                  }
                }
              }
            }
            n434 = local write "stepMotor/ECU"(w22) -> ()
          }
          frame #1 {
            n435 = shared-variable "我的电脑\\Modbus.lvlib\\工步号"() -> (w842:u16)  [unwired: 1 in, 1 out]
            n436 = local read "stepMotor/ECU"() -> (w846:string)
            n437 = local read "布尔"() -> (w844:bool)
            n438 = Equal?(x=w842, y=i8 -100) -> (x = y?=w845:bool)
            n439 = Or(x=w845, y=w844) -> (x .or. y?=w843:bool)
            n440 = case shown="真" w843 {
              tunnel: [w849 w852] -> w847
              tunnel: w846 -> [w849 w851]
              frame False {
              }
              frame True {
                (unwired) "10"
                n441 = shared-variable "我的电脑\\Modbus.lvlib\\工步号"() -> (w850:u16)  [unwired: 1 in, 1 out]
                n442 = local write "布尔"(TRUE ("布尔")) -> ()
                n443 = Equal?(x=w850, y=i8 0) -> (x = y?=w854:bool)
                n444 = call "AlarmInsert.vi"("消息名"="复位中" ("string_5")) -> ()  [unwired: 11 in]
                n445 = case shown="真" w854 {
                  tunnel: [w857 "10"] -> w852
                  tunnel: w851 -> [w857 _]
                  frame False {
                  }
                  frame True {
                    n446 = local write "布尔"(FALSE ("布尔")) -> ()
                  }
                }
              }
            }
            n447 = local write "stepMotor/ECU"(w847) -> ()
          }
          frame #2 {
            n448 = global read "全局 3.vi" "stop"() -> (w860:bool)
            n449 = Wait (ms)(milliseconds to wait=u32 10 ("等待时间（毫秒）")) -> ()  [unwired: 1 out]
          }
        }
      }
    }
    frame #2 {
      n450 = global read "resultShow.vi" "runMode"() -> (w863:refnum<vi>)
      n451 = property class="Bool"(reference=w863, "Value"=FALSE ("m")) -> ()  [unwired: 1 in, 2 out]
    }
  }
  n452 = local read "毫秒计时值"() -> (w7:u32)
  n453 = Tick Count (ms)() -> (millisecond timer value=w2:u32)
  n454 = Subtract(x=w2, y=w7) -> (x-y=w3:u32)
  n455 = Divide(x=w3, y=u32 1000) -> (x/y=w5:dbl)
  n456 = Tick Count (ms)() -> (millisecond timer value=w9:u32)
  n457 = To Time Stamp(1:w5) -> (0:w6:timestamp)
  n458 = local write "毫秒计时值"(w9) -> ()
  n459 = Format Date/Time String(seconds (now)=w6) -> (date/time string=w8:string)  [unwired: 2 in]
  n460 = call "AlarmInsert.vi"("takesTime"=w8, "消息名"="完成取回工件！" ("string_5")) -> ()  [unwired: 10 in]
  n461 = disable-structure shown="禁用" {
    frame Disabled {
      n462 = call "TCP_write.vi"("写入数据"=i8 13) -> ()  [unwired: 11 in]
      n463 = call "AlarmInsert.vi"("消息名"="请放回检具1" ("string_5")) -> ()  [unwired: 11 in]
    }
    frame Enabled {
    }
  }
